vi "Launch Single Assert Display.vi"(8 "error in (no error)":errorcluster, 10 "Assert UID":string, 11 "Main Display in":refnum<class "Main Display.lvclass">) -> (0 "error out":errorcluster, 3 "Main Display out":refnum<class "Main Display.lvclass">)   [LabVIEW 2016]
uses:
  <vilib>/ActorFramework/Actor/Actor.lvclass
  Main Display.lvclass
  C:/Users/ukhornp/Documents/Projects/actor_assert_api/Core/Base UI Component/Base UI Component/Base UI Component.lvclass
  C:/Users/ukhornp/Documents/Projects/actor_assert_api/Core/Base UI Actor/Base UI Actor/Base UI Actor.lvclass
  C:/Program Files (x86)/National Instruments/LabVIEW 2016/vi.lib/ActorFramework/Actor/Actor.lvclass
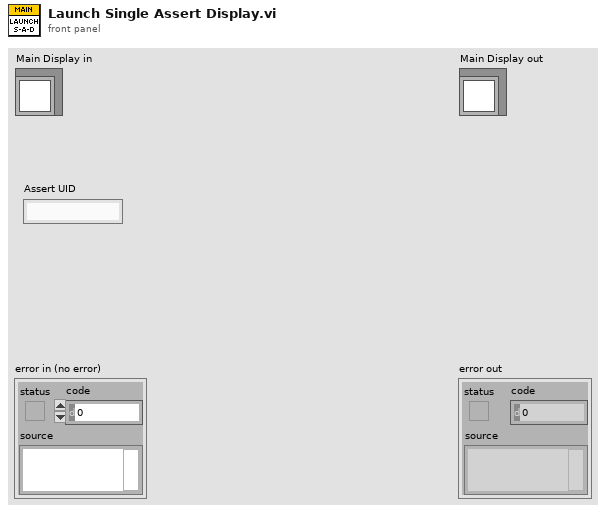
[diagram p1: front panel]
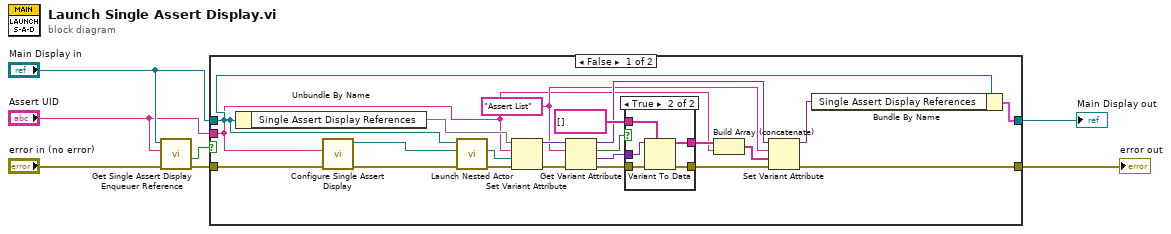
[diagram p0: block diagram]
diagram:
  n1 = call "Get Single Assert Display Enqueuer Reference.vi"("error in (no error)"="error in (no error)", "Assert UID"="Assert UID", "Main Display in"="Main Display in") -> ("error out"=w4:errorcluster, "Assert Display Active?"=w6:bool)  [unwired: 6 in, 1 out]
  n2 = case shown="False" w6 {
    tunnel: "Main Display in" -> [w23 w37]
    tunnel: w4 -> [w27 w38]
    tunnel: "Assert UID" -> [w8 _]
    tunnel: [w13 w38] -> w2
    tunnel: [w21 w37] -> w1
    frame False {
      w10 = "Assert List" ("name")
      n3 = Unbundle By Name(w23) -> ("Single Assert Display References"=w26)
      n4 = call "Configure Single Assert Display.vi"("error in (no error)"=w27, "Assert UID"=w8) -> ("error out"=w28:errorcluster, "Single Assert Display out"=w29:refnum<class "Single Assert Display.lvclass">)  [unwired: 8 in]
      n5 = call <vilib>:"Launch Nested Actor.vi"("error in (no error)"=w28, "Nested Actor"=w29, "Caller Actor in"=w23) -> ("error out"=w24:errorcluster, "Nested Actor's Enqueuer"=w25:refnum<class "Message Enqueuer.lvclass">)  [unwired: 6 in, 1 out]
      n6 = Set Variant Attribute(Variant=w26, name=w8, value=w25, error in=w24) -> (Variant out=w19:variant, error out=w22:errorcluster)  [unwired: 1 out]
      n7 = Get Variant Attribute(Variant=w19, name=w10, error in=w22) -> (duplicate Variant=w12:variant, found=w15:bool, value=w17:variant, error out=w20:errorcluster)  [unwired: 1 in]
      n8 = case shown="True" w15 {
        tunnel: w20 -> [w31 w36]
        tunnel: [w31 w35] -> w18
        tunnel: w17 -> [_ w34]
        tunnel: string[] [] -> [w30 w33]
        tunnel: [w30 w32] -> w14
        frame False {
        }
        frame True {
          n9 = Variant To Data(error in=w36, type=w33, Variant=w34) -> (data=w32:string[], error out=w35:errorcluster)
        }
      }
      n10 = Build Array (concatenate)(w14, w8) -> (w9:string[])
      n11 = Set Variant Attribute(Variant=w12, name=w10, value=w9, error in=w18) -> (Variant out=w11:variant, error out=w13:errorcluster)  [unwired: 1 out]
      n12 = Bundle By Name(cluster=w23, "Single Assert Display References"=w11) -> (w21:cluster{})
    }
    frame True {
    }
  }
  "error out" <- w2
  "Main Display out" <- w1
